vi "Read Network Slave.vi"(8 "error in (no error)":errorcluster, 11 "Modbus Slave in":refnum<class "Modbus Slave.lvclass">) -> (0 "error out":errorcluster, 2 "Network Slave":refnum<class "Network Slave.lvclass">, 3 "Modbus Slave out":refnum<class "Modbus Slave.lvclass">)   [LabVIEW 2021, in "Modbus Slave.lvclass"]
uses:
  Modbus Slave.lvclass
  Network Protocol/Network Slave/Network Slave.lvclass
  Modbus Slave.lvclass/Modbus Slave.ctl
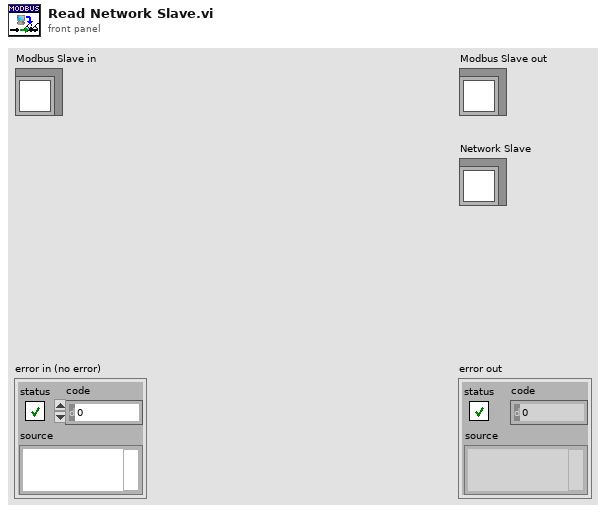
[diagram p1: front panel]
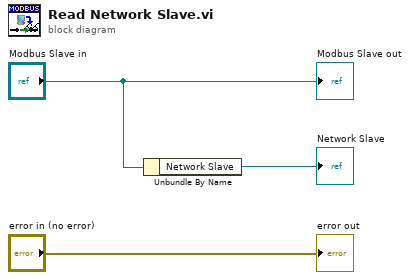
[diagram p0: block diagram]
diagram:
  n1 = Unbundle By Name("Modbus Slave in") -> ("Network Slave"=→"Network Slave":refnum<class "Network Slave.lvclass">)
  "error out" <- "error in (no error)"
  "Modbus Slave out" <- "Modbus Slave in"
